vi "Create.vi"(7 "Direction":T1, 8 "error in (no error)":errorcluster, 9 "Custom Config Data":u8[](array[numeric]), 10 "Name":string, 11 "CIFFIFO in":refnum<class "CIF_CIPC_Fifo_U8.lvclass">) -> (0 "error out":errorcluster, 3 "CIFFIFO out":refnum<class "CIF_CIPC_Fifo_U8.lvclass">)   [LabVIEW 2021, in "CIF_CIPC_Fifo_U8.lvclass"]
uses:
  CIF_CIPC_Fifo_U8.lvclass
  CIFChannels/Typedef/Direction.ctl
  D:/dev/Packages/CIF_Channels_Core/src/CIFChannels/CIFChannels.lvclass
  D:/dev/Packages/CIF_Channels_Core/src/CIPC_Channels/CIF_CIPC_Chan/CIF_CIPC_Chn.lvclass
  <vilib>/CIF Foundation/CIF Utilities/Statistics/I64/Stats_I64_CIF_U.lvclass/Stats_I64_CIF_U.ctl
  CIFChannels/Typedef/Channel State.ctl
  CIFChannels/Typedef/Disconnect Behavior.ctl
  CIFChannels/CIFChannels.lvclass/CIFChannels.ctl
  ChannelCommon/typedef/Channel Pattern.ctl
  CIF_CIPC_Chan/Typedef/Buffer Configuration Data.ctl
  <vilib>/CIF Foundation/CIF CIPC/TypeDefs/Backpressure References.ctl
  CIF_CIPC_Chan/CIF_CIPC_Chn.lvclass/CIF_CIPC_Chn.ctl
  CIF_CIPC_Fifo_U8.lvclass/CIF_CIPC_Fifo_U8.ctl
  35849dc3-58aa-4d75-b906-fe3df34869a7.vi
  CIFChannels/Accessors/Write Pattern.vi
  CIF_CIPC_Chan/Accessors/Write Buffer Configuration.vi
  CIF_CIPC_Chan/Accessors/Write CIPC Channel.vi
  9be4d617-3037-4515-bcea-2a1e3727d04e.vi
  CIFChannels/Accessors/Write Channel State.vi
  CIFChannels/Accessors/Write Channel Benchmark.vi
  CIFChannels/Accessors/Write Flatten Benchmark.vi
  CIFChannels/SubVIs/Get Type from Class.vi
  ChannelCommon/Utilities/Unflatten FIFO Config.vi
  CIFChannels/Utilities/Apply Flags.vi
  CIFChannels/Accessors/Write Type.vi
  CIFChannels/Accessors/Write Channel Class.vi
  CIFChannels/Accessors/Write Direction.vi
  CIFChannels/Accessors/Write Tag Disconnect Behavior.vi
  CIFChannels/Accessors/Write Name.vi
  CIFChannels/Accessors/Write Custom Config Data.vi
  35849dc3-58aa-4d75-b906-fe3df34869a7.vi/bd07d5d9-1209-45ad-b636-9e9ab86132fb.vi
  <vilib>/CIF Foundation/CIF CIPC/SubVIs/Check Error.vi
  <vilib>/CIF Foundation/CIF CIPC/SubVIs/Get dll Path.vi
  9be4d617-3037-4515-bcea-2a1e3727d04e.vi/bd07d5d9-1209-45ad-b636-9e9ab86132fb.vi
  9be4d617-3037-4515-bcea-2a1e3727d04e.vi/1e2c93d0-55b0-4d6c-a9da-21395a664279.vi
  <vilib>/CIF Foundation/CIF CIPC/SubVIs/Get Backpressure Name.vi
  9be4d617-3037-4515-bcea-2a1e3727d04e.vi/7bb13226-97f3-4dcb-9346-06ec631a2876.vi
  <vilib>/CIF Foundation/CIF Utilities/DataTypes/Flatten Unflatten/Unflatten U64.vi
  ChannelCommon/Utilities/Expand FIFO Flags.vi
  9be4d617-3037-4515-bcea-2a1e3727d04e.vi/1e2c93d0-55b0-4d6c-a9da-21395a664279.vi/49b3dd2d-4579-4089-b72e-3f0875c862f2.vi
  <vilib>/CIF Foundation/CIF CIPC/SubVIs/Notify Of New Write.vi
  <vilib>/CIF Foundation/CIF CIPC/SubVIs/Get Element Write Position.vi
  <vilib>/Utility/LVClass/Get LV Class Name.vi
  <vilib>/CIF Foundation/CIF CIPC/SubVIs/Get Element Description Variant.vi
  <vilib>/Utility/error.llb/Trim Whitespace.vi
  <vilib>/string/Create NI GUID.vi
  <vilib>/Utility/error.llb/Error Cluster From Error Code.vi
  <vilib>/CIF Foundation/CIF CIPC/SubVIs/Get Element Info Variant.vi
  <vilib>/CIF Foundation/CIF Utilities/Statistics/I64/Stats_I64_CIF_U.lvclass
  CIFChannels/CIFChannels.lvclass
  ChannelCommon/ChannelCommon.lvlib
  <vilib>/CIF Foundation/CIF CIPC/CIF_NI_CIPC.lvlib
  CIF_CIPC_Chan/CIF_CIPC_Chn.lvclass
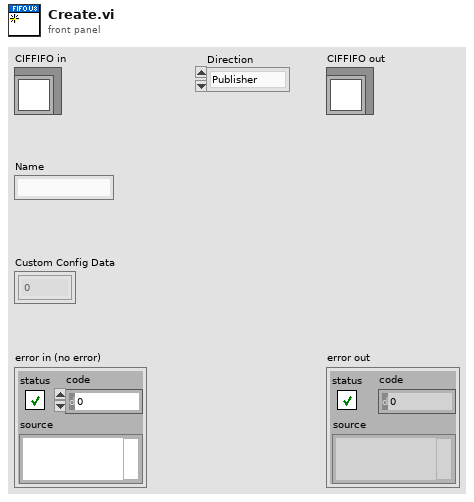
[diagram p1: front panel]
types:
  T1 = typedef "CIFChannels.lvclass/Direction.ctl" = enum16{"Publisher", "Subscriber"}
  T2 = typedef "CIFChannels.lvclass/Channel State.ctl" = enum16{"Creating", "Disconnected", "Connecting", "Connected", "Destroyed"}
  T3 = typedef "CIFChannels.lvclass/Disconnect Behavior.ctl" = enum16{"Default value", "Last value", "Error with default"}
  T4 = typedef "ChannelCommon.lvlib/Channel Pattern.ctl" = enum16{"Unknown", "Tag", "FIFO", "MultiFIFO", "BackpressureFIFO"}
  T5 = typedef "CIF_CIPC_Chn.lvclass/Buffer Configuration Data.ctl" = cluster{"Total Size":u32, "Read Size":u32, "Read Offset":u32, "CIPC BP References":T6, "Override CIPC Name":string, "Encoder Data":string}
  T6 = typedef "CIF_NI_CIPC.lvlib/Backpressure References.ctl" = cluster{"CIPC Reference":u64, "CIPC BP Reference":u64}
  T7 = typedef "CIF_NI_CIPC.lvlib/Encoder Info.ctl" = cluster{"Name":string, "Version":i32, "Data":string}
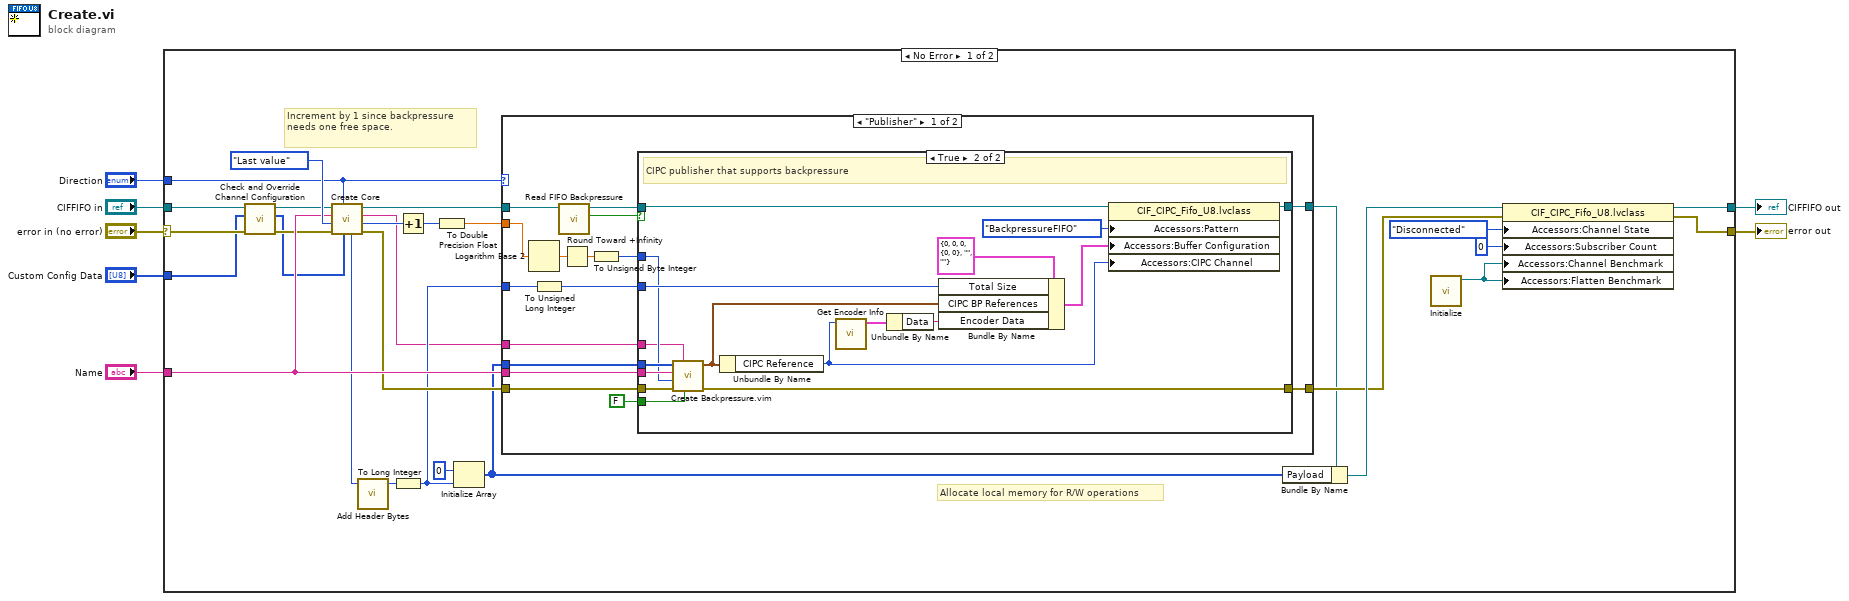
[diagram p0: block diagram]
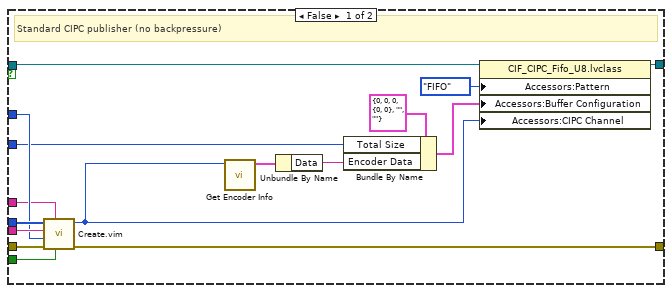
[diagram p2: hidden frame]
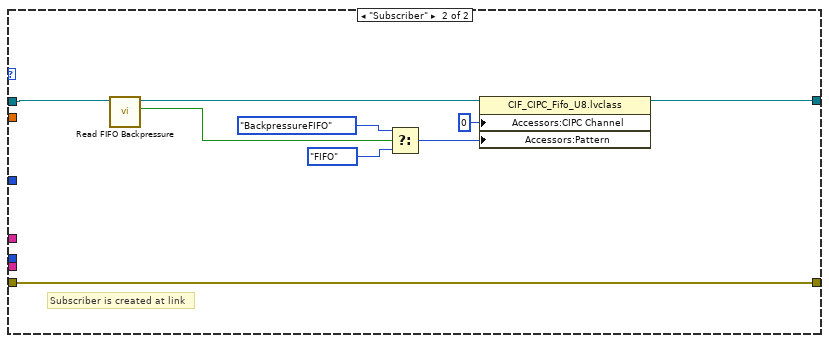
[diagram p3: hidden frame]
diagram:
  n1 = case shown="No Error" "error in (no error)" {
    selector: "error in (no error)" -> [w24 w95]
    tunnel: [w34 w95] -> w6
    tunnel: [w29 w94] -> w1
    tunnel: "CIFFIFO in" -> [w25 w94]
    tunnel: "Name" -> [w33 _]
    tunnel: "Direction" -> [w28 _]
    tunnel: "Custom Config Data" -> [w21 _]
    frame No Error {
      # "Increment by 1 since backpressure needs one free space."
      # "Allocate local memory for R/W operations"
      n2 = call-dynamic "Check and Override Channel Configuration.vi"("error in (no error)"=w24, "Custom Config Data in"=w21, "CIFFIFO in"=w25) -> ("error out"=w22:errorcluster, "Custom Config Data out"=w20:u8[], "CIFFIFO out"=w23:refnum<class "CIF_CIPC_Fifo_U8.lvclass">)  [unwired: 6 in]
      n3 = call "Create Core.vi"("Custom Config Data"=w20, "Direction"=w28, "error in (no error)"=w22, "Disconnect Behavior"=Disconnect_Behavior."Last value", "Name"=w33, "CIFChannels in"=w23) -> ("error out"=w32:errorcluster, "Messages"=w12:u64, "Channel Type"=w10:string, "CIFChannels out"=w16:refnum<class "CIF_CIPC_Fifo_U8.lvclass">, "Bytes/Msg"=w19:u64)  [unwired: 1 in]
      n4 = call "Add Header Bytes.vi"("Bytes/Msg"=w19) -> ("Bytes/Msg with header"=w15:u64)  [unwired: 3 in]
      n5 = To Long Integer(number=w15) -> (32bit integer=w14:i32)
      n6 = Increment(x=w12) -> (x+1=w11:u64)
      n7 = To Double Precision Float(number=w11) -> (double precision float=w17:dbl)
      n8 = Initialize Array(u8 0 ("Numeric"), w14) -> (w18:u8[])
      n9 = case shown="\"Publisher\"" w28 {
        tunnel: w33 -> [w48 _]
        tunnel: w32 -> [w50 w93]
        tunnel: [w51 w93] -> w30
        tunnel: w17 -> [w45 _]
        tunnel: w18 -> [w47 _]
        tunnel: w16 -> [w42 w90]
        tunnel: w14 -> [w39 _]
        tunnel: [w37 w92] -> w13
        tunnel: w10 -> [w36 _]
        frame "Publisher" {
          n10 = Logarithm Base 2(1:w45) -> (0:w46:dbl)
          n11 = To Unsigned Long Integer(number=w39) -> (unsigned 32bit integer=w38:u32)
          n12 = call "Read FIFO Backpressure.vi"("CIFChannels in"=w42) -> ("Backpressure"=w40:bool, "CIFChannels out"=w41:refnum<class "CIF_CIPC_Fifo_U8.lvclass">)  [unwired: 8 in, 1 out]
          n13 = Round Toward +Infinity(x=w46) -> (ceil(x): smallest int >= x=w44:dbl)
          n14 = To Unsigned Byte Integer(number=w44) -> (unsigned 8bit integer=w43:u8)
          n15 = case shown="True" w40 {
            tunnel: [w67 w73] -> w51
            tunnel: w50 -> [w66 w74]
            tunnel: FALSE ("Prepend Array Size") -> [w65 w77]
            tunnel: w48 -> [w64 w76]
            tunnel: w47 -> [w63 w78]
            tunnel: w43 -> [w62 w75]
            tunnel: w41 -> [w61 w84]
            tunnel: w38 -> [w59 w82]
            tunnel: [w55 w79] -> w37
            tunnel: w36 -> [w54 w70]
            frame False {
              # "Standard CIPC publisher (no backpressure)"
              n16 = call "Create.vim"("Prepend Array Size"=w65, "Description"=w54, "error in (no error)"=w66, "Buffer Size N (2^N)"=w62, "Name in"=w64, "Data Type"=w63) -> ("error out"=w67:errorcluster, "CIPC Reference"=w56:u64)  [unwired: 2 in, 2 out]
              n17 = call <vilib>:"Get Encoder Info.vi"("CIPC Reference"=w56) -> ("Encoder Info"=w58:T7)  [unwired: 9 in, 1 out]
              n18 = Unbundle By Name(w58) -> ("Data"=w57:string)
              n19 = Bundle By Name(cluster=T5 {"Total Size"=0, "Read Size"=0, "Read Offset"=0, "CIPC BP References"={"CIPC Reference"=0, "CIPC BP Reference"=0}, "Override CIPC Name"="", "Encoder Data"=""} ("Buffer Configuration"), "Total Size"=w59, "Encoder Data"=w57) -> (w53:T5)
              n20 = property class="CIF_CIPC_Fifo_U8.lvclass"(reference=w61, "Accessors:Pattern"=Channel_Pattern."FIFO" ("Pattern"), "Accessors:Buffer Configuration"=w53, "Accessors:CIPC Channel"=w56) -> (reference out=w55:refnum<class "CIF_CIPC_Fifo_U8.lvclass">)  [unwired: 1 in, 1 out]
            }
            frame True {
              # "CIPC publisher that supports backpressure"
              n21 = call "Create Backpressure.vim"("Prepend Array Size"=w77, "Description"=w70, "error in (no error)"=w74, "Buffer Size N (2^N)"=w75, "Name in"=w76, "Data Type"=w78) -> ("error out"=w73:errorcluster, "CIPC BP References"=w71:T6)  [unwired: 2 in, 2 out]
              n22 = Unbundle By Name(w71) -> ("CIPC Reference"=w72:u64)
              n23 = call <vilib>:"Get Encoder Info.vi"("CIPC Reference"=w72) -> ("Encoder Info"=w81:T7)  [unwired: 9 in, 1 out]
              n24 = Unbundle By Name(w81) -> ("Data"=w80:string)
              n25 = Bundle By Name(cluster=T5 {"Total Size"=0, "Read Size"=0, "Read Offset"=0, "CIPC BP References"={"CIPC Reference"=0, "CIPC BP Reference"=0}, "Override CIPC Name"="", "Encoder Data"=""} ("Buffer Configuration"), "Total Size"=w82, "CIPC BP References"=w71, "Encoder Data"=w80) -> (w69:T5)
              n26 = property class="CIF_CIPC_Fifo_U8.lvclass"(reference=w84, "Accessors:Pattern"=Channel_Pattern."BackpressureFIFO" ("Pattern"), "Accessors:Buffer Configuration"=w69, "Accessors:CIPC Channel"=w72) -> (reference out=w79:refnum<class "CIF_CIPC_Fifo_U8.lvclass">)  [unwired: 1 in, 1 out]
            }
          }
        }
        frame "Subscriber" {
          # "Subscriber is created at link"
          n27 = call "Read FIFO Backpressure.vi"("CIFChannels in"=w90) -> ("Backpressure"=w88:bool, "CIFChannels out"=w89:refnum<class "CIF_CIPC_Fifo_U8.lvclass">)  [unwired: 8 in, 1 out]
          n28 = Select(t=Channel_Pattern."BackpressureFIFO" ("Pattern"), s=w88, f=Channel_Pattern."FIFO" ("Pattern")) -> (s? t:f=w85:T4)
          n29 = property class="CIF_CIPC_Fifo_U8.lvclass"(reference=w89, "Accessors:CIPC Channel"=u64 0 ("CIPC Channel"), "Accessors:Pattern"=w85) -> (reference out=w92:refnum<class "CIF_CIPC_Fifo_U8.lvclass">)  [unwired: 1 in, 1 out]
        }
      }
      n30 = Bundle By Name(cluster=w13, "Payload"=w18) -> (w31:refnum<class "CIF_CIPC_Fifo_U8.lvclass">)
      n31 = call <vilib>:"Initialize.vi"() -> ("Stats_I64_CIF_U out"=w26:refnum<class "Stats_I64_CIF_U.lvclass">)  [unwired: 10 in, 1 out]
      n32 = property class="CIF_CIPC_Fifo_U8.lvclass"(reference=w31, error in=w30, "Accessors:Channel State"=Channel_State."Disconnected" ("Channel State"), "Accessors:Subscriber Count"=u32 0 ("Subscriber Count"), "Accessors:Channel Benchmark"=w26, "Accessors:Flatten Benchmark"=w26) -> (reference out=w29:refnum<class "CIF_CIPC_Fifo_U8.lvclass">, error out=w34:errorcluster)
    }
    frame Error {
    }
  }
  "error out" <- w6
  "CIFFIFO out" <- w1
